vi "setAcqFormat.vi"(6 "Delay between send and receive [ms]":i32=100, 8 "error in (no error)":errorcluster, 9 "format":i32, 10 "number of ROIs":i32, 11 "CCD in":refnum<class "CCD.lvclass">) -> (0 "error out":errorcluster, 1 "ID":i32, 2 "results-JSON string":string, 3 "CCD out":refnum<class "CCD.lvclass">)   [LabVIEW 2023, in "CCD.lvclass"]
doc: "Sets the acquisition format and the number of ROIs (Regions of Interest) or areas. This command will remove all previously defined ROIs. After using this command, the ccd_setRoi command should be used to define each ROI.\n\nparameter description\nnumberOfRois Integer. Number of ROIs (Regions of Interest / areas)\nformat Integer. The acquisition format.\n0 = Spectra\n1 = Image\n2 = Crop*\n3 = Fast Kinetics*\n* Note: The Crop (2) and Fast Kinetics (3) acquisition formats are not supported by every CCD."
uses:
  CCD.lvclass
  CCD.lvclass/CCD.ctl
  20f7d3bd-08ac-4524-9bed-df36c1da25a0.vi
  GenericDevice/GenericDevice.lvclass
  9c26a383-523e-4ef9-a52a-706f8f4d1e65.vi
  1afe4a3d-b8bf-4f9d-9cc3-ba347473a4dc.vi
panel:
  # "Connector Pane"
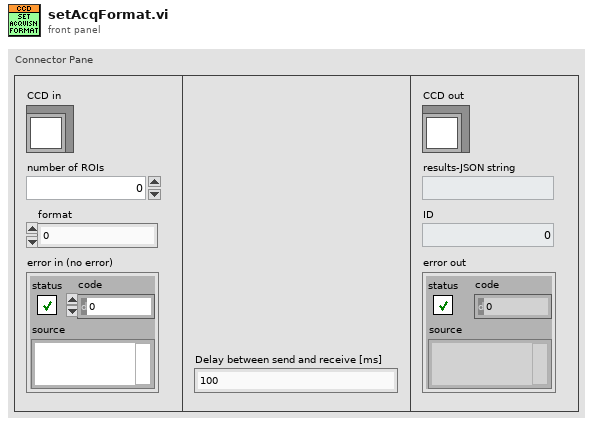
[diagram p1: front panel]
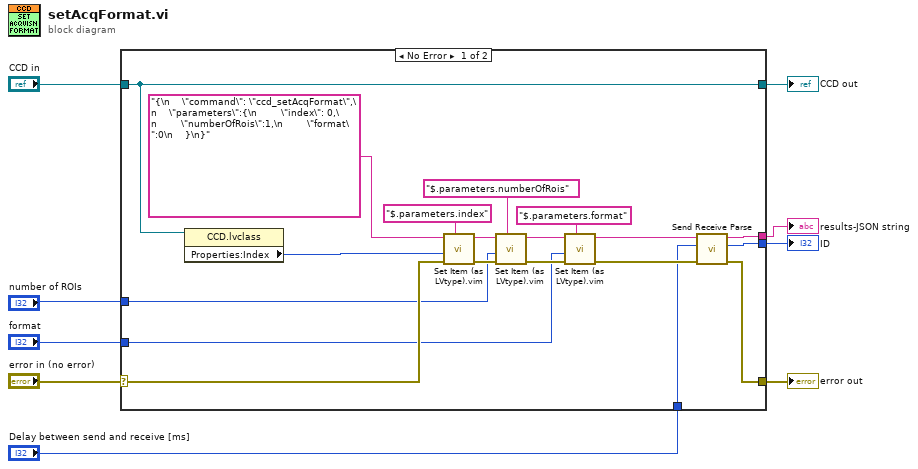
[diagram p0: block diagram]
diagram:
  n1 = case shown="No Error" "error in (no error)" {
    selector: "error in (no error)" -> [w24 w30]
    tunnel: [w15 w30] -> w8
    tunnel: [w26 w29] -> w6
    tunnel: "CCD in" -> [w26 w29]
    tunnel: "number of ROIs" -> [w16 _]
    tunnel: [w14 _] -> w4
    tunnel: [w13 _] -> w3
    tunnel: "Delay between send and receive [ms]" -> [w11 _]
    tunnel: "format" -> [w10 _]
    frame No Error {
      n2 = property class="CCD.lvclass"(reference=w26) -> ("Properties:Index"=w25:i32)  [unwired: 1 in, 2 out]
      n3 = call "Set Item (as LVtype).vim"("$Path or Item Name"="$.parameters.index", "error in (no error)"=w24, "Anything"=w25, "JSON"="{\n    \"command\": \"ccd_setAcqFormat\",\n    \"parameters\":{\n        \"index\": 0,\n        \"numberOfRois\":1,\n        \"format\":0\n    }\n}") -> ("error out"=w21:errorcluster, "<JSON>"=w22:string)  [unwired: 4 in, 1 out]
      n4 = call "Set Item (as LVtype).vim"("$Path or Item Name"="$.parameters.numberOfRois", "error in (no error)"=w21, "Anything"=w16, "JSON"=w22) -> ("error out"=w19:errorcluster, "<JSON>"=w20:string)  [unwired: 4 in, 1 out]
      n5 = call "Set Item (as LVtype).vim"("$Path or Item Name"="$.parameters.format", "error in (no error)"=w19, "Anything"=w10, "JSON"=w20) -> ("error out"=w18:errorcluster, "<JSON>"=w12:string)  [unwired: 4 in, 1 out]
      n6 = call "Send Receive Parse.vi"("error in"=w18, "Delay between send and receive [ms]"=w11, "<JSON>"=w12) -> ("error out"=w15:errorcluster, "ID"=w13:i32, "results-JSON string"=w14:string)  [unwired: 6 in]
    }
    frame Error {
    }
  }
  "error out" <- w8
  "CCD out" <- w6
  "results-JSON string" <- w4
  "ID" <- w3
